vi "H5Sset_extent_simple.vi"(6 "error in (no error)":errorcluster, 7 "Maximum Dimensions (unlimited)":u64[](array[numeric]), 8 "Dimensions":u64[](array[numeric]), 9 "HDF5 Space Ref":T1) -> (0 "error out":errorcluster, 3 "HDF5 Ref":T1)   [LabVIEW 2017]
doc: "Sets or resets the size of an existing dataspace."
uses:
  <vilib>/UPVI/lvhdf5/library.llb/HDF5 Ref.ctl
  <vilib>/UPVI/lvhdf5/hdf5.dll
panel:
  # "LVHDF5 Toolkit\nCopyright (c) 2005-2013 by Jason D. Sommerville\nCopyright (c) 2014 by UPVI, LLC.\n\nThis use and distribution of this file is governed by the terms found in \nLICENSE.txt distributed with this toolkit and installed at\n <user.lib>\\_lvhdf5\\LICENSE.txt"
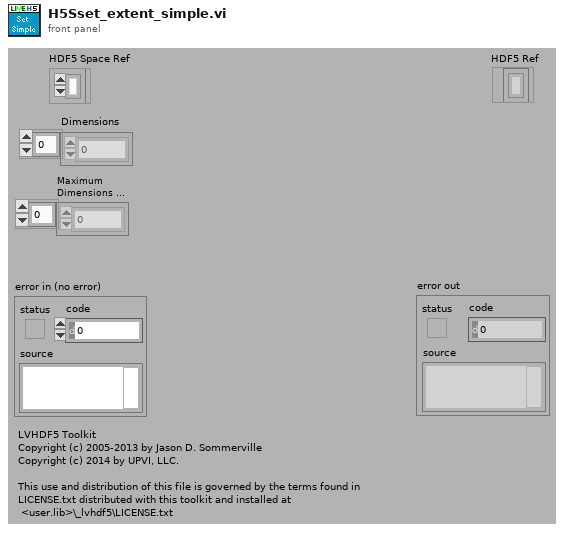
[diagram p1: front panel]
types:
  T1 = typedef "HDF5 Ref.ctl" = refnum<k1>
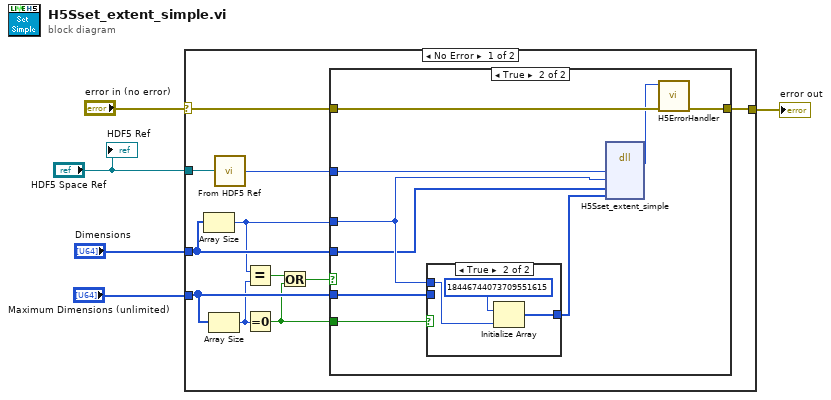
[diagram p0: block diagram]
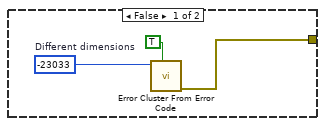
[diagram p2: hidden frame]
diagram:
  n1 = case shown="No Error" "error in (no error)" {
    selector: "error in (no error)" -> [w16 w33]
    tunnel: [w15 w33] -> w4
    tunnel: "Dimensions" -> [w13 _]
    tunnel: "Maximum Dimensions (unlimited)" -> [w14 _]
    tunnel: "HDF5 Space Ref" -> [w7 _]
    frame No Error {
      n2 = Array Size(array=w13) -> (size(s)=w11:i32)
      n3 = Array Size(array=w14) -> (size(s)=w12:i32)
      n4 = call <vilib>:"From HDF5 Ref.vi"("HDF5 Ref"=w7) -> ("I32"=w6:i32)
      n5 = Equal?(x=w11, y=w12) -> (x = y?=w10:bool)
      n6 = Equal To 0?(x=w12) -> (x = 0?=w9:bool)
      n7 = Or(x=w10, y=w9) -> (x .or. y?=w8:bool)
      n8 = case shown="True" w8 {
        tunnel: w16 -> [_ w28]
        tunnel: [w19 w27] -> w15
        tunnel: w9 -> [_ w26]
        tunnel: w14 -> [_ w25]
        tunnel: w13 -> [_ w21]
        tunnel: w11 -> [_ w23]
        tunnel: w6 -> [_ w22]
        frame False {
          w17 = -23033  # Different dimensions
          n9 = call <vilib>:"Error Cluster From Error Code.vi"("show call chain? (False)"=TRUE, "error code (0)"=w17) -> ("error out"=w19:errorcluster)  [unwired: 7 in]
        }
        frame True {
          n10 = case shown="True" w26 {
            tunnel: w23 -> [_ w31]
            tunnel: [w29 w30] -> w20
            tunnel: w25 -> [w29 _]
            frame False {
            }
            frame True {
              n11 = Initialize Array(u64 18446744073709551615, w31) -> (w30:u64[])
            }
          }
          n12 = dll-call lib="C:/Program Files/National Instruments/LabVIEW 2017/vi.lib/UPVI/lvhdf5/hdf5.dll" fn="H5Sset_extent_simple"("space_id"=w22, "rank"=w23, "dims"=w21, "maxdims"=w20) -> ("return type"=w24:i32)  [unwired: 7 in, 2 out]
          n13 = call <vilib>:"H5ErrorHandler.vi"("error in (no error)"=w28, "herr_t"=w24) -> ("error out"=w27:errorcluster)  [unwired: 3 in, 4 out]
        }
      }
    }
    frame Error {
    }
  }
  "error out" <- w4
  "HDF5 Ref" <- "HDF5 Space Ref"
